vi "Test Print Label.vi"() -> ()   [LabVIEW 2018]
panel:
  in  "stop":bool
  in  "Print":bool
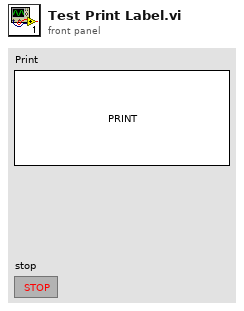
[diagram p1: front panel]
types:
  T1 = cluster{"appended path":path, "appended path":path, "appended path":path, "appended path":path}
  T2 = cluster{"appended path":string, "appended path":string, "appended path":string, "appended path":string}
  T3 = cluster{"ME79 Pass":refnum<k7>, "ME79 Fail":refnum<k7>, "ME74 Pass":refnum<k7>, "ME74 Fail":refnum<k7>, "App Ref Out":refnum<k7>, "ActiveX Ref Out":refnum<k7>}
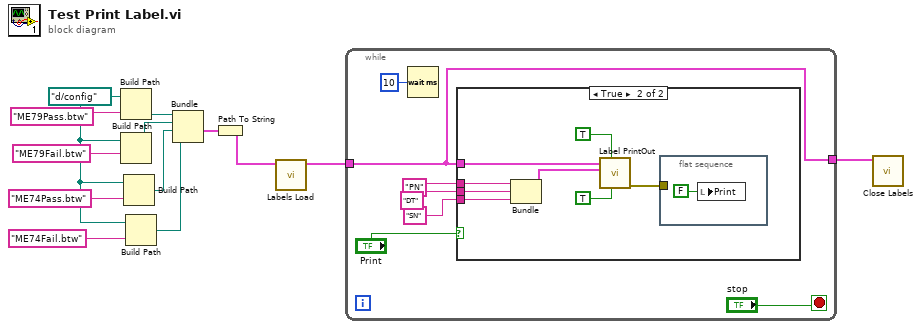
[diagram p0: block diagram]
diagram:
  w9 = path "d:/config" ("base path")
  n1 = Build Path(base path=w9, name or relative path="ME79Pass.btw") -> (appended path=w8:path)
  n2 = Build Path(base path=w9, name or relative path="ME79Fail.btw") -> (appended path=w7:path)
  n3 = Build Path(base path=w9, name or relative path="ME74Pass.btw") -> (appended path=w6:path)
  n4 = Build Path(base path=w9, name or relative path="ME74Fail.btw") -> (appended path=w5:path)
  n5 = Bundle("appended path"=w8, "appended path"=w7, "appended path"=w6, "appended path"=w5) -> (w4:T1)  [unwired: 1 in]
  n6 = Path To String(path=w4) -> (string=w3:T2)
  n7 = call "Labels Load.vi"("Labels"=w3) -> ("File Open Reference out"=w2:T3)  [unwired: 9 in, 1 out]
  n8 = while {
    tunnel: w2 -> [w14]
    tunnel: [w14] -> w1
    stop <- "stop" stop-if-true
    n9 = Wait (ms)(milliseconds to wait=u32 10) -> ()  [unwired: 1 out]
    n10 = case shown="True" "Print" {
      tunnel: w14 -> [_ w28]
      tunnel: "PN" -> [_ w26]
      tunnel: "DT" -> [_ w25]
      tunnel: "SN" -> [_ w24]
      frame False {
      }
      frame True {
        n11 = Bundle(w26, w25, w24) -> (w23:cluster{string, string, string})  [unwired: 1 in]
        n12 = call "Label PrintOut.vi"("Model (F-ME74)"=TRUE, "Label Print Pass/Fail (F-Fail)"=TRUE, "Pass Data"=w23, "Labels Reference In"=w28) -> ("error out"=w21:errorcluster)  [unwired: 7 in]
        n13 = flat-sequence {
          tunnel: w21 -> [_]
          frame #0 {
            n14 = local write "Print"(FALSE ("Print")) -> ()
          }
        }
      }
    }
  }
  n15 = call "Close Labels.vi"("Labels Reference In"=w1) -> ()  [unwired: 10 in, 1 out]
